vi "Edit_Raw_DF.vi"(5 "Edit Raw Data Header Info":bool, 7 "New Values In":string[](array[string])=[""], 8 "New Chs In":string[](array[string])=[""], 9 "Data filename":path) -> (0 "Filetype":string, 1 "Original values":string[](array[string]), 3 "Data filename out":path, 4 "File Not Changed?":bool)   [LabVIEW 2010]
uses:
  Globals/Constants_global.vi
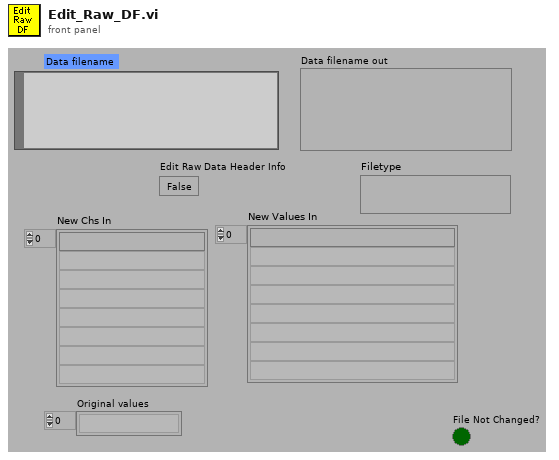
[diagram p1: front panel]
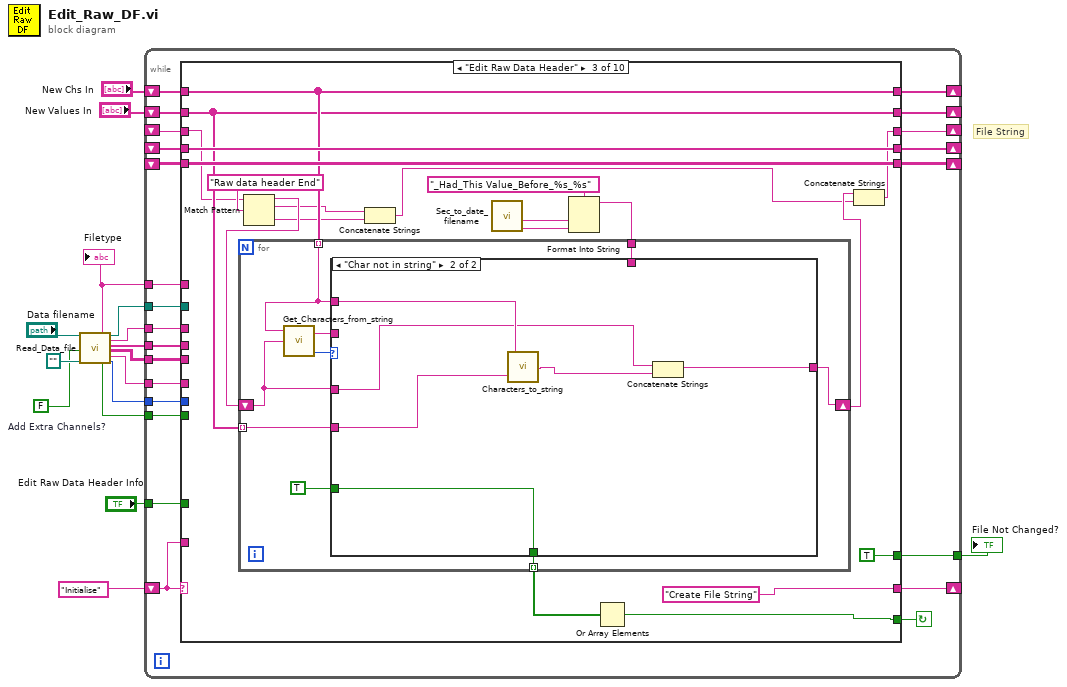
[diagram p0: block diagram]
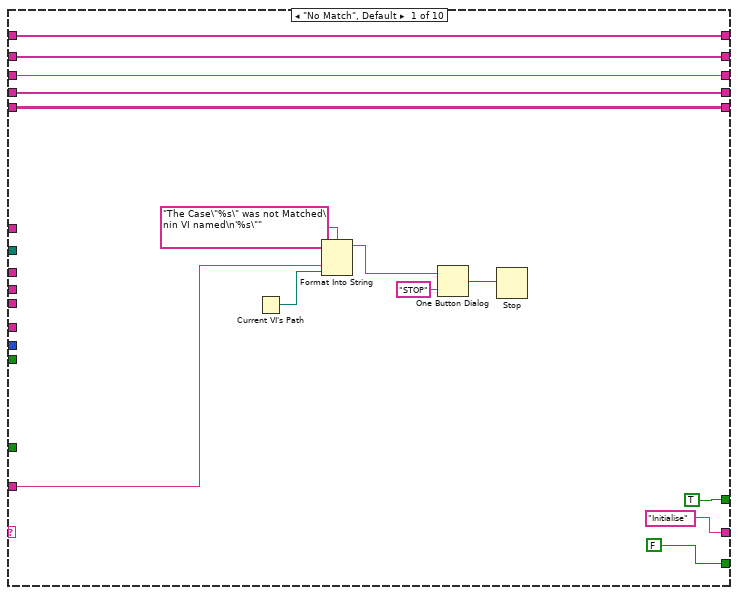
[diagram p2: hidden frame]
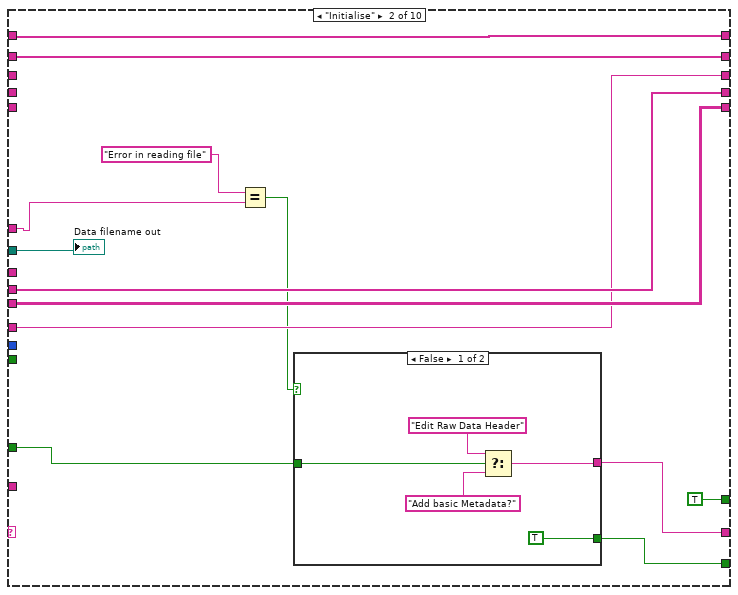
[diagram p3: hidden frame]
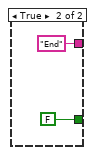
[diagram p4: hidden frame]
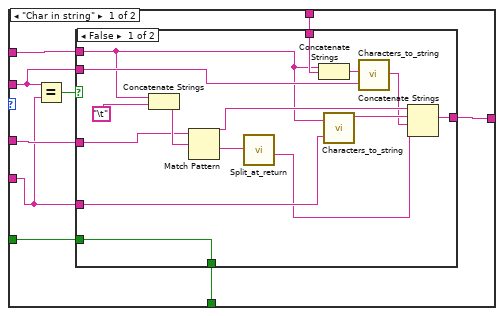
[diagram p5: hidden frame]
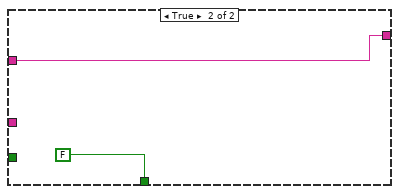
[diagram p6: hidden frame]
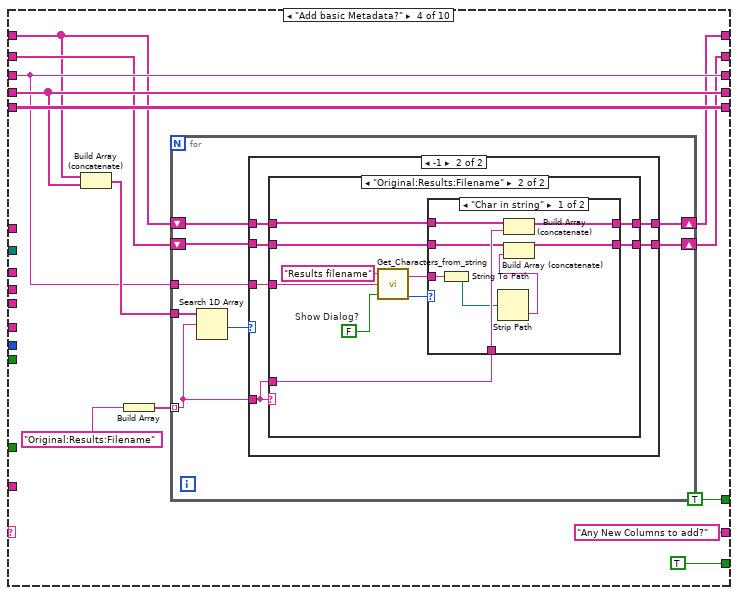
[diagram p7: hidden frame]
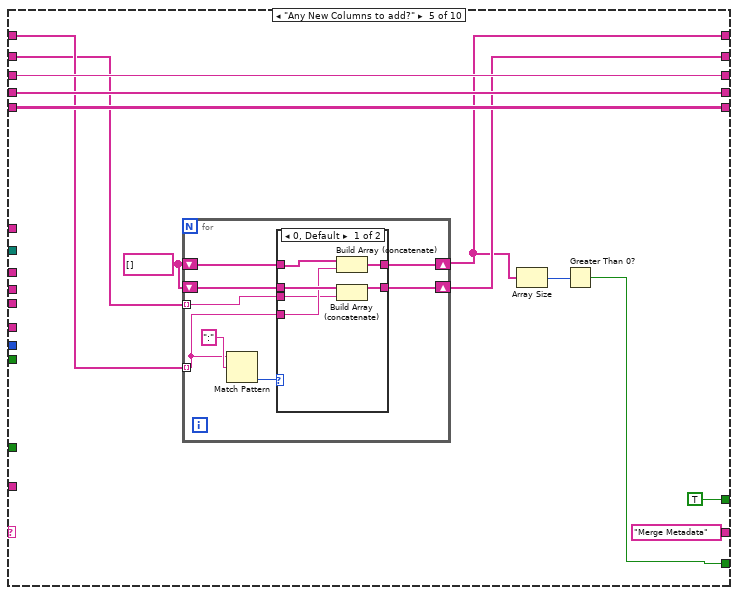
[diagram p11: hidden frame]
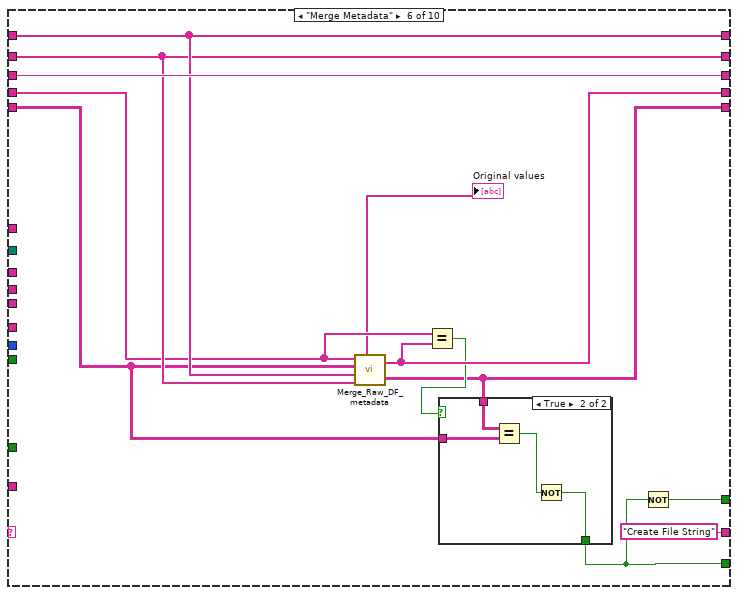
[diagram p13: hidden frame]
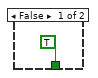
[diagram p14: hidden frame]
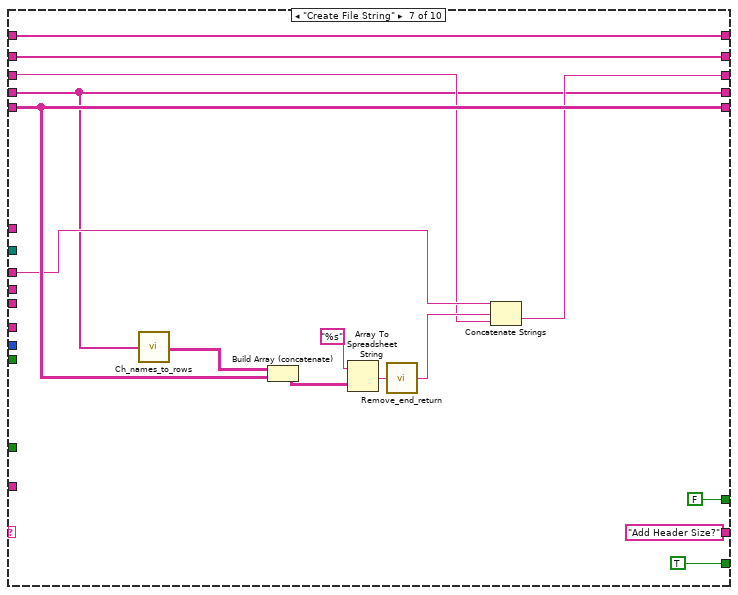
[diagram p15: hidden frame]
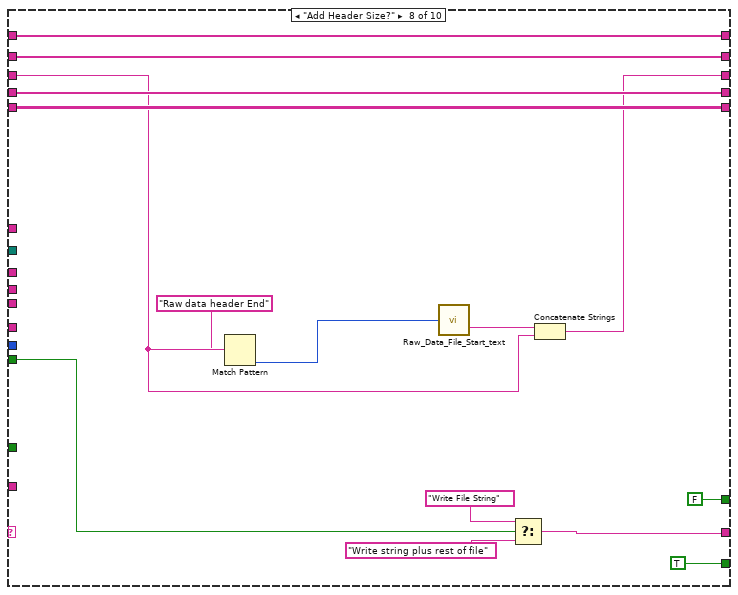
[diagram p16: hidden frame]
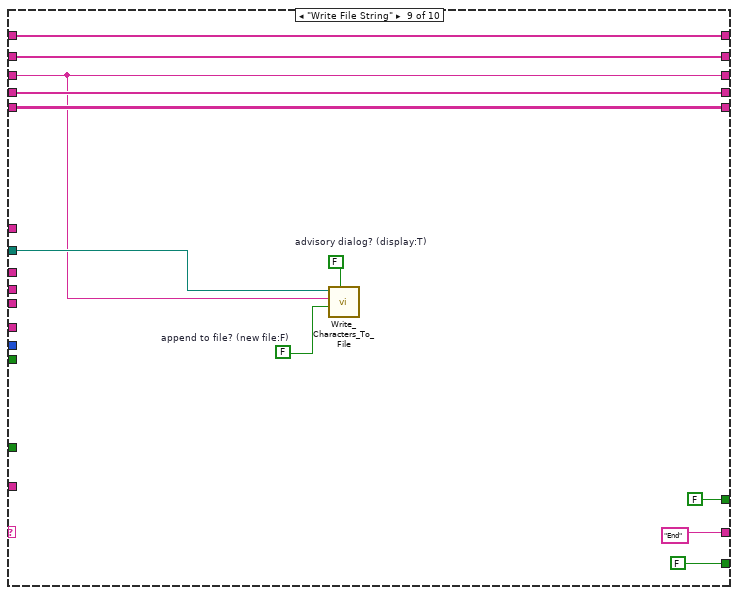
[diagram p17: hidden frame]
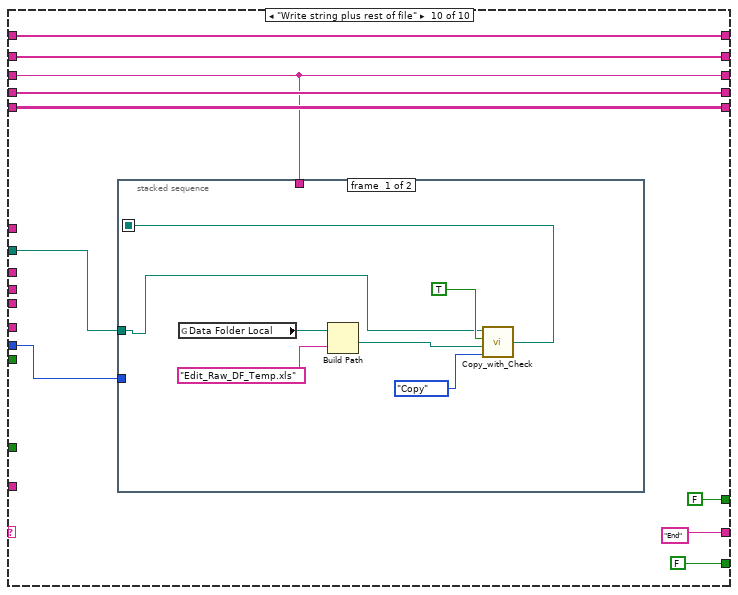
[diagram p18: hidden frame]
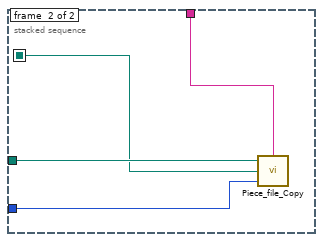
[diagram p19: hidden frame]
diagram:
  w14 = FALSE  # Add Extra Channels?
  # "File String"
  n1 = call "Read_Data_file.vi"("Results file"="Data filename", "Add Extra Channels?"=w14, "Template File"=path "") -> ("Filetype"=w9:string, "EOF?"=w7:bool, "Results file Out"=w12:path, "String Before"=w8:string, "Ch names Out"=w11:string[], "Channel Values Out"=w10:string[][], "String After"=w6:string, "mark after read (chars.)"=w5:i32)  [unwired: 2 in, 7 out]
  "Filetype" <- w9
  n2 = while {
    tunnel: "Edit Raw Data Header Info" -> [w18]
    shift-left: "New Values In" -> [w20]
    shift-right: [w19] -> _
    shift-left: "New Chs In" -> [w22]
    shift-right: [w21] -> _
    tunnel: w5 -> [w23]
    tunnel: w6 -> [w24]
    tunnel: w7 -> [w25]
    tunnel: w8 -> [w26]
    tunnel: w9 -> [w27]
    tunnel: w10 -> [w28]
    tunnel: w11 -> [w29]
    tunnel: w12 -> [w30]
    shift-left: _ -> [w31]
    shift-right: [w35] -> _
    shift-left: _ -> [w32]
    shift-right: [w34] -> _
    shift-left: _ -> [w33]
    shift-right: [w36] -> _
    shift-left: "Initialise" -> [w37]
    shift-right: [w38] -> _
    tunnel: [w17] -> w1
    stop <- w39 continue-if-true
    n3 = case shown="\"Edit Raw Data Header\"" w37 {
      tunnel: [FALSE w54 w75 TRUE w193 w216 TRUE TRUE FALSE FALSE] -> w39
      tunnel: ["Initialise" w58 "Create File String" ("f") "Any New Columns to add?" "Merge Metadata" ("f") "Create File String" ("f") "Add Header Size?" ("f") w254 "End" "End"] -> w38
      tunnel: w37 -> [w48 _ _ _ _ _ _ _ _ _]
      tunnel: [w45 w61 w78 w140 w197 w225 w238 w252 w266 w276] -> w36
      tunnel: [w43 w62 w93 w146 w196 w219 w240 w258 w269 w279] -> w35
      tunnel: [w44 w63 w92 w143 w195 w222 w232 w259 w270 w280] -> w34
      tunnel: w33 -> [w45 _ w84 w140 w197 w225 w234 w253 w266 w276]
      tunnel: w32 -> [w44 _ w92 w143 w195 w221 w232 w259 w270 w280]
      tunnel: w31 -> [w43 _ w93 w146 w196 w218 w240 w258 w269 w279]
      tunnel: w30 -> [_ w66 _ _ _ _ _ _ w267 w277]
      tunnel: w29 -> [_ w63 _ _ _ _ _ _ _ _]
      tunnel: w28 -> [_ w62 _ _ _ _ _ _ _ _]
      tunnel: w27 -> [_ w56 _ _ _ _ _ _ _ _]
      tunnel: w26 -> [_ _ _ _ _ _ w239 _ _ _]
      tunnel: w25 -> [_ _ _ _ _ _ _ w255 _ _]
      tunnel: w24 -> [_ w61 _ _ _ _ _ _ _ _]
      tunnel: w23 -> [_ _ _ _ _ _ _ _ _ w275]
      tunnel: w22 -> [w42 w65 w87 w136 w189 w224 w236 w251 w263 w274]
      tunnel: [w42 w65 w87 w139 w187 w224 w236 w251 w263 w274] -> w21
      tunnel: w20 -> [w41 w64 w86 w137 w188 w223 w235 w250 w262 w273]
      tunnel: [w41 w64 w86 w138 w190 w223 w235 w250 w262 w273] -> w19
      tunnel: w18 -> [_ w59 _ _ _ _ _ _ _ _]
      tunnel: [TRUE TRUE TRUE TRUE TRUE w215 FALSE FALSE FALSE FALSE] -> w17
      frame "No Match", Default {
        n4 = Current VI's Path() -> (path=w47:path)
        n5 = Format Into String(format string="The Case\"%s\" was not Matched\nin VI named\n'%s\"" ("Format String"), w48, w47) -> (resulting string=w51:string)  [unwired: 2 in, 1 out]
        n6 = One Button Dialog(message=w51, button name ("OK")="STOP") -> (true=w49:bool)
        n7 = Stop(stop? (T)=w49) -> ()
      }
      frame "Initialise" {
        n8 = Equal?(x="Error in reading file", y=w56) -> (x = y?=w55:bool)
        n9 = case shown="False" w55 {
          tunnel: w59 -> [w69 _]
          tunnel: [w68 "End"] -> w58
          tunnel: [TRUE FALSE] -> w54
          frame False {
            n10 = Select(t="Edit Raw Data Header", s=w69, f="Add basic Metadata?") -> (s? t:f=w68:string)
          }
          frame True {
          }
        }
        "Data filename out" <- w66
      }
      frame "Edit Raw Data Header" {
        n11 = Match Pattern(string=w84, regular expression="Raw data header End") -> (before substring=w83:string, match substring=w82:string, after substring=w81:string)  [unwired: 2 out]
        n12 = Concatenate Strings(w82, w81) -> (w79:string)
        n13 = call "Sec_to_date_filename.vi"() -> ("Day"=w89:string, "Time"=w74:string)  [unwired: 1 in, 2 out]
        n14 = Format Into String(format string="_Had_This Value_Before_%s_%s" ("Format String"), w89, w74) -> (resulting string=w90:string)  [unwired: 2 in, 1 out]
        n15 = for {
          shift-right: [w97] -> w80
          shift-left: w83 -> [w99]
          tunnel: w87 -> [w100] mode=indexing
          tunnel: w86 -> [w98] mode=indexing
          tunnel: w90 -> [w96]
          tunnel: [w95] -> w76 mode=indexing
          n16 = call "Get_Characters_from_string.vi"("Input string"=w99, "Variable name"=w100) -> ("Status"=w102:enum16{"Char in string", "Char not in string"}, "Value"=w101:string)  [unwired: 1 in]
          n17 = case shown="\"Char not in string\"" w102 {
            tunnel: w100 -> [w109 w134]
            tunnel: w98 -> [w108 w133]
            tunnel: [w110 w132] -> w97
            tunnel: w99 -> [w111 w131]
            tunnel: w101 -> [w106 _]
            tunnel: w96 -> [w105 _]
            tunnel: [w104 w129] -> w95
            tunnel: TRUE -> [w103 w129]
            frame "Char in string" {
              n18 = Equal?(x=w106, y=w108) -> (x = y?=w107:bool)
              n19 = case shown="False" w107 {
                tunnel: w111 -> [w124 w128]
                tunnel: [w122 w128] -> w110
                tunnel: w108 -> [w121 _]
                tunnel: w109 -> [w115 _]
                tunnel: w106 -> [w117 _]
                tunnel: w105 -> [w116 _]
                tunnel: [w112 FALSE] -> w104
                tunnel: w103 -> [w112 _]
                frame False {
                  n20 = Concatenate Strings(w115, "\t") -> (w125:string)
                  n21 = Match Pattern(string=w124, regular expression=w125) -> (before substring=w119:string, after substring=w123:string)  [unwired: 3 out]
                  n22 = call "Split_at_return.vi"("String"=w123) -> ("after substring"=w118:string)  [unwired: 1 in, 3 out]
                  n23 = Concatenate Strings(w115, w116) -> (w114:string)
                  n24 = call "Characters_to_string.vi"("Characters to write"=w121, "Label for characters"=w115) -> ("Output string"=w120:string)
                  n25 = call "Characters_to_string.vi"("Characters to write"=w117, "Label for characters"=w114) -> ("Output string"=w113:string)
                  n26 = Concatenate Strings(w119, w120, w113, w118) -> (w122:string)
                }
                frame True {
                }
              }
            }
            frame "Char not in string" {
              n27 = call "Characters_to_string.vi"("Characters to write"=w133, "Label for characters"=w134) -> ("Output string"=w130:string)
              n28 = Concatenate Strings(w131, w130) -> (w132:string)
            }
          }
        }
        n29 = Or Array Elements(Boolean array=w76) -> (logical OR=w75:bool)
        n30 = Concatenate Strings(w80, w79) -> (w78:string)
      }
      frame "Add basic Metadata?" {
        n31 = Build Array (concatenate)(w136, w143) -> (w141:string[])
        n32 = Build Array("Original:Results:Filename") -> (w142:string[])
        n33 = for {
          tunnel: w142 -> [w153] mode=indexing
          tunnel: w141 -> [w154]
          shift-right: [w152] -> w139
          shift-left: w136 -> [w151]
          shift-right: [w149] -> w138
          shift-left: w137 -> [w150]
          tunnel: w140 -> [w148]
          n34 = Search 1D Array(1D array=w154, element=w153) -> (index of element=w155:i32)  [unwired: 1 out]
          n35 = case shown="-1" w155 {
            tunnel: w153 -> [_ w158]
            tunnel: [w157 w163] -> w152
            tunnel: w151 -> [w157 w162]
            tunnel: w150 -> [w156 w161]
            tunnel: [w156 w160] -> w149
            tunnel: w148 -> [_ w159]
            frame 0, Default {
            }
            frame -1 {
              n36 = case shown="\"Original:Results:Filename\"" w158 {
                tunnel: [w165 w169] -> w163
                tunnel: w162 -> [w165 w171]
                tunnel: w161 -> [w164 w167]
                tunnel: [w164 w166] -> w160
                tunnel: w159 -> [_ w174]
                tunnel: w158 -> [_ w170]
                frame "Other", Default {
                }
                frame "Original:Results:Filename" {
                  w173 = FALSE  # Show Dialog?
                  n37 = call "Get_Characters_from_string.vi"("Show Dialog?"=w173, "Input string"=w174, "Variable name"="Results filename") -> ("Status"=w172:enum16{"Char in string", "Char not in string"}, "Value"=w168:string)
                  n38 = case shown="\"Char in string\"" w172 {
                    tunnel: w171 -> [w183 w185]
                    tunnel: w170 -> [w182 _]
                    tunnel: [w181 w185] -> w169
                    tunnel: w168 -> [w180 _]
                    tunnel: w167 -> [w178 w184]
                    tunnel: [w177 w184] -> w166
                    frame "Char in string" {
                      n39 = String To Path(string=w180) -> (path=w179:path)
                      n40 = Strip Path(path=w179) -> (name=w176:string)  [unwired: 1 out]
                      n41 = Build Array (concatenate)(w183, w182) -> (w181:string[])
                      n42 = Build Array (concatenate)(w178, w176) -> (w177:string[])
                    }
                    frame "Char not in string" {
                    }
                  }
                }
              }
            }
          }
        }
      }
      frame "Any New Columns to add?" {
        w191 = string[] []
        n43 = for {
          tunnel: w189 -> [w199] mode=indexing
          shift-right: [w200] -> w187
          shift-left: w191 -> [w203]
          shift-right: [w202] -> w190
          shift-left: w191 -> [w201]
          tunnel: w188 -> [w198] mode=indexing
          n44 = Match Pattern(string=w199, regular expression=":") -> (offset past match=w204:i32)  [unwired: 4 out]
          n45 = case shown="0, Default" w204 {
            tunnel: [w208 w213] -> w200
            tunnel: w203 -> [w211 w213]
            tunnel: [w209 w212] -> w202
            tunnel: w201 -> [w210 w212]
            tunnel: w199 -> [w207 _]
            tunnel: w198 -> [w206 _]
            frame 0, Default {
              n46 = Build Array (concatenate)(w211, w207) -> (w208:string[])
              n47 = Build Array (concatenate)(w210, w206) -> (w209:string[])
            }
            frame -1 {
            }
          }
        }
        n48 = Array Size(array=w187) -> (size(s)=w194:i32)
        n49 = Greater Than 0?(x=w194) -> (x > 0?=w193:bool)
      }
      frame "Merge Metadata" {
        n50 = call "Merge_Raw_DF_metadata.vi"("New Values In"=w223, "New Chs In"=w224, "Orig Values In"=w218, "Orig Chs In"=w221) -> ("Channel Values Out"=w219:string[][], "Ch names Out"=w222:string[], "Original values"=→"Original values":string[])  [unwired: 1 in]
        n51 = Equal?(x=w221, y=w222) -> (x = y?=w220:bool)
        n52 = case shown="True" w220 {
          tunnel: [TRUE w227] -> w216
          tunnel: w219 -> [_ w230]
          tunnel: w218 -> [_ w229]
          frame False {
          }
          frame True {
            n53 = Equal?(x=w230, y=w229) -> (x = y?=w228:bool)
            n54 = Not(x=w228) -> (.not. x?=w227:bool)
          }
        }
        n55 = Not(x=w216) -> (.not. x?=w215:bool)
      }
      frame "Create File String" {
        n56 = call "Ch_names_to_rows.vi"("Channel Names"=w232) -> ("3 Row names"=w231:string[][])
        n57 = Build Array (concatenate)(w231, w240) -> (w241:string[][])
        n58 = Array To Spreadsheet String(array=w241, 3:"%s" ("format string")) -> (spreadsheet string=w243:string)  [unwired: 1 out]
        n59 = call "Remove_end_return.vi"("Input string"=w243) -> ("Output string"=w244:string)
        n60 = Concatenate Strings(w239, w244, w234) -> (w238:string)
      }
      frame "Add Header Size?" {
        n61 = Match Pattern(string=w253, regular expression="Raw data header End") -> (offset past match=w247:i32)  [unwired: 4 out]
        n62 = call "Raw_Data_File_Start_text.vi"("Header length"=w247) -> ("Start String"=w246:string)
        n63 = Select(t="Write File String", s=w255, f="Write string plus rest of file") -> (s? t:f=w254:string)
        n64 = Concatenate Strings(w246, w253) -> (w252:string)
      }
      frame "Write File String" {
        w265 = FALSE  # append to file? (new file:F)
        w268 = FALSE  # advisory dialog? (display:T)
        n65 = call "Write_Characters_To_File.vi"("file path (dialog if empty)"=w267, "advisory dialog? (display:T)"=w268, "character string"=w266, "append to file? (new file:F)"=w265) -> ()  [unwired: 1 in, 4 out]
      }
      frame "Write string plus rest of file" {
        n66 = stacked-sequence {
          seq-local: [w282 _] -> [_ w290]
          tunnel: w277 -> [w283 w291]
          tunnel: w276 -> [_ w292]
          tunnel: w275 -> [_ w289]
          frame #0 {
            n67 = global read "Constants_global.vi" "Data Folder Local"() -> (w287:path)
            n68 = Build Path(base path=w287, name or relative path="Edit_Raw_DF_Temp.xls") -> (appended path=w284:path)
            n69 = call "Copy_with_Check.vi"("Mode"=enum16{"Move", "Copy"}."Copy", "Target Path"=w284, "Variable Target?"=TRUE, "Source Path"=w283) -> ("Pathname Out"=w282:path)
          }
          frame #1 {
            n70 = call "Piece_file_Copy.vi"("File Start String"=w292, "Start to copy file at:"=w289, "Source File"=w290, "Target File"=w291) -> ()  [unwired: 1 out]
          }
        }
      }
    }
  }
  "File Not Changed?" <- w1
